vi "ACC_LabVIEW_Write_Example.vi"() -> ()   [LabVIEW 2014, in "ACC_LabVIEW.lvlib"]
doc: "Example for using the \"write\" method."
uses:
  ACC_LabVIEW.lvlib
  DataConverter/LabVIEW2AccData_Float64.vi
  DataConverter/LabVIEW2AccData_Float32.vi
  DataConverter/Acc2LabVIEWData_UWord.vi
  DataConverter/Acc2LabVIEWData_Float32.vi
panel:
  in  "VirtAcc":i32=1
  out "FieldI":sgl
  out "FieldS":sgl
  out "Status":bool
  in  "Desired FieldS":sgl=-0.3
  in  "Desired Status":bool
  out "error out":errorcluster
  in  "Nomenklatur":string="GTR1KYB"
  # "Please notice:\n\nA read-action wil work every time on every device. But to perform a \"write\" or \"call\" , you need \nto be registered inside the \"right.xml\" file of the nameserver.\nTo get this managed, ask Solveigh Matthies from the BEL - department."
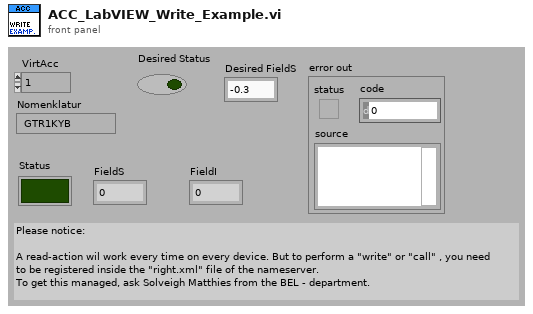
[diagram p1: front panel]
types:
  T1 = typedef "ACC_LabVIEW.lvlib/ACC_LabVIEW_Container.ctl" = cluster{"Data Type":T2, "String":string, "Double":dbl}
  T2 = typedef "ACC_LabVIEW.lvlib/ACC_LabVIEW_DataTypes.ctl" = enum16{"SByte (8Bit Int signed)", "UByte (8Bit int unsigned)", "SWord (16Bit Int signed)", "UWord (16Bit Int unsigned)", "SLong (32Bit Int signed)", "ULong (32Bit Int unsigned)", "Float32 (float)", "Float64 (double)", "String"}
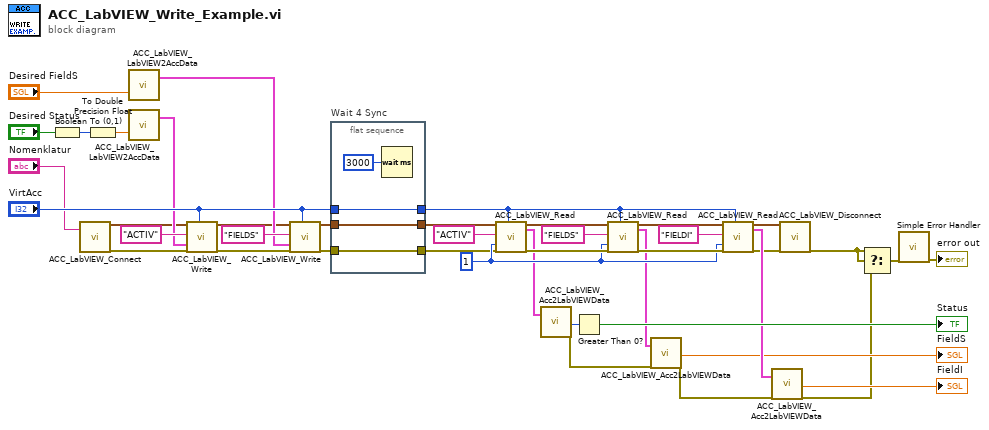
[diagram p0: block diagram]
diagram:
  w34 = u32 1 ("#of expected Elements in \"Acc_Data_Out\"")
  n1 = Boolean To (0,1)(Boolean="Desired Status") -> (0, 1=w32:i16)
  n2 = call "ACC_LabVIEW_Connect.vi"("Nomenklatur"="Nomenklatur") -> ("DeviceReferenceOut"=w11:cluster{"ID":u32}, "error out"=w1:errorcluster)  [unwired: 17 in]
  n3 = To Double Precision Float(number=w32) -> (double precision float=w25:dbl)
  n4 = call-poly "ACC_LabVIEW_LabVIEW2AccData.vi"("Value"="Desired FieldS") -> ("Acc_Data_Out"=w24:T1[])  [unwired: 18 in]
  n5 = call-poly "ACC_LabVIEW_LabVIEW2AccData.vi"("Value"=w25) -> ("Acc_Data_Out"=w26:T1[])  [unwired: 18 in]
  n6 = call "ACC_LabVIEW_Write.vi"("DeviceReferenceIn"=w11, "Propname"="ACTIV", "Acc_Data_In"=w26, "error in (no error)"=w1, "VirtAcc"="VirtAcc") -> ("DeviceReferenceOut"=w10:cluster{"ID":u32}, "error out"=w41:errorcluster)  [unwired: 12 in, 1 out]
  n7 = call "ACC_LabVIEW_Write.vi"("DeviceReferenceIn"=w10, "Propname"="FIELDS" ("Propname 2"), "Acc_Data_In"=w24, "error in (no error)"=w41, "VirtAcc"="VirtAcc") -> ("DeviceReferenceOut"=w7:cluster{"ID":u32}, "error out"=w30:errorcluster)  [unwired: 12 in, 1 out]
  n8 = flat-sequence "Wait 4 Sync" {
    tunnel: w30 -> [w46]
    tunnel: [w46] -> w29
    tunnel: "VirtAcc" -> [w45]
    tunnel: [w45] -> w27
    tunnel: [w43] -> w8
    tunnel: w7 -> [w43]
    frame #0 {
      n9 = Wait (ms)(milliseconds to wait=u32 3000) -> ()  [unwired: 1 out]
    }
  }
  n10 = call "ACC_LabVIEW_Read.vi"("DeviceReferenceIn"=w8, "Propname"="ACTIV", "#of expected Elements in \"Acc_Data_Out\""=w34, "error in (no error)"=w29, "VirtAcc"=w27) -> ("DeviceReferenceOut"=w6:cluster{"ID":u32}, "Acc_Data_Out"=w22:T1[], "error out"=w38:errorcluster)  [unwired: 10 in, 2 out]
  n11 = call-poly "ACC_LabVIEW_Acc2LabVIEWData.vi"("Acc_Data_In"=w22) -> ("Value"=w21:u32, "error out"=w20:errorcluster)  [unwired: 16 in, 1 out]
  n12 = Greater Than 0?(x=w21) -> (x > 0?=→"Status":bool)
  n13 = call "ACC_LabVIEW_Read.vi"("DeviceReferenceIn"=w6, "Propname"="FIELDS", "#of expected Elements in \"Acc_Data_Out\""=w34, "error in (no error)"=w38, "VirtAcc"=w27) -> ("DeviceReferenceOut"=w5:cluster{"ID":u32}, "Acc_Data_Out"=w19:T1[], "error out"=w37:errorcluster)  [unwired: 10 in, 2 out]
  n14 = call-poly "ACC_LabVIEW_Acc2LabVIEWData.vi"("Acc_Data_In"=w19, "error in"=w20) -> ("Value"=→"FieldS":sgl, "error out"=w17:errorcluster)  [unwired: 15 in, 1 out]
  n15 = call "ACC_LabVIEW_Read.vi"("DeviceReferenceIn"=w5, "Propname"="FIELDI", "#of expected Elements in \"Acc_Data_Out\""=w34, "error in (no error)"=w37, "VirtAcc"=w27) -> ("DeviceReferenceOut"=w4:cluster{"ID":u32}, "Acc_Data_Out"=w18:T1[], "error out"=w3:errorcluster)  [unwired: 10 in, 2 out]
  n16 = call-poly "ACC_LabVIEW_Acc2LabVIEWData.vi"("Acc_Data_In"=w18, "error in"=w17) -> ("Value"=→"FieldI":sgl, "error out"=w14:errorcluster)  [unwired: 15 in, 1 out]
  n17 = call "ACC_LabVIEW_Disconnect.vi"("DeviceReferenceIn"=w4, "error in (no error)"=w3) -> ("error out"=w2:errorcluster)  [unwired: 17 in]
  n18 = Select(t=w2, s=w2, f=w14) -> (s? t:f=w13:errorcluster)
  n19 = call <vilib>:"Simple Error Handler.vi"("error in (no error)"=w13) -> ("error out"=→"error out":errorcluster)  [unwired: 4 in, 4 out]
